vi "calibrate_tip.vi"() -> ()   [LabVIEW 2014]
uses:
  <vilib>/Analysis/Matrix/Datatypes/RealMatrix.ctl
  asap/labview/testing/calibration_task.ctl
  asap/labview/testing/cal_display_mode.ctl
  asap/labview/testing/probe_calibration.ctl
  <vilib>/Platform/TimedLoop/XDataNode/timing_clust.ctl
  <vilib>/Platform/TimedLoop/XDataNode/nitl_modes.ctl
  <vilib>/Platform/TimedLoop/XDataNode/wakeup.ctl
  testing/probe_point.ctl
  testing/pose_source.ctl
  <vilib>/gmath/NumericalOptimization/stopping criteria.ctl
  <vilib>/Analysis/baseanly.llb/A x Vector.vi
  initialization/micron_globals.vi
  <vilib>/gmath/NumericalOptimization/Downhill Simplex.vi
  <vilib>/Platform/TimedLoop/XDataNode/XDataNode.xnode
  <vilib>/Platform/TimedLoop/XDataNode/XDNodeRunTimeDep.lvlib
  <vilib>/Analysis/NI_AALBase.lvlib
  <vilib>/gmath/NI_Gmath.lvlib
  <vilib>/Analysis/Matrix/NI_Matrix.lvlib
panel:
  in  "Reference points 2":T1 format="%#.0f"
  in  "Valid override":bool
  out "status":bool
  out "Invalid data":bool
  out "Light triad error":dbl[](array[numeric]) format="%#.0f"
  out "Triad error":dbl
  in  "Save solution":bool
  in  "Clear all ref points":bool
  in  "Reference points":T1 format="%#.0f"
  in  "Calibration task":T2
  in  "Selector":bool[](array[boolean])
  out "Residuals":dbl[](array[numeric]) format="%#.0f"
  in  "Clear all":bool
  out "New point":dbl[](array[numeric]) format="%#.0f"
  in  "Save point":bool
  out "Number of poses":i32 format="%22.0f"
  out "Current point":dbl[](array[numeric]) format="%#.0f"
  out "RMS error":dbl format="%#22.0f"
  in  "Start calibration":bool
  out "Display mode":T3
  out "Light positions":sgl[][](array[numeric]) format="%#.2f"
  out "New light positions":sgl[][](array[numeric]) format="%#.2f"
  in  "Initialize light pos":bool
  in  "z offset":sgl=2262.0
  out "Calibration poses":dbl[][][](array[numeric])
  in  "stop":bool
  # "Point calibration (pivot)"
  # "(mm)"
  # "Position status"
  # "Three point calibrations"
  # "Handle"
  # "Tip"
  # "(mm)"
  # "(mm)"
  # "To calibrate the tip or RCM offset, position Micron in serveral different poses, keeping the desired calibration point (tip or RCM) fixed, but vary on all three of the rotational axes.  To record a pose, click \"Add pose\" or use the foot pedal to trigger a trace cycle.  The tool should be held still during the 0.2 sec data collection.  This can be done either fixtured or handheld, with or without cancellation. \n\nRecording least four poses is recommended.  RMS error should be <200 mm if fixtured, or ~ 1mm handheld.  You can use the \"Selector\" to remove poses with high residuals from the calibration.  Observe the sensitivity of  \"New point\" to adding and removing a pose from the estimate.  \"Save point\" stores this calibration into the running system.  To make it persistent, save it into the default configuration."
  # "Tip calibration requires a pivot calibration at each of three fiducial points on that part (either handle or tip.)  Fixture the probe, collect one pose, then press \"Initialize\".  Then do three pivot procedures (as for tip offset calibration.)  \"Save Point\" adds the measured location to the \"Reference Points\". Observe \"Triad error\" as a santity check. Finally, press \"Save solution.\"  Once tip lights have been calibrated and saved, the handle lights only need to be initialized (according to \"z offset\")."
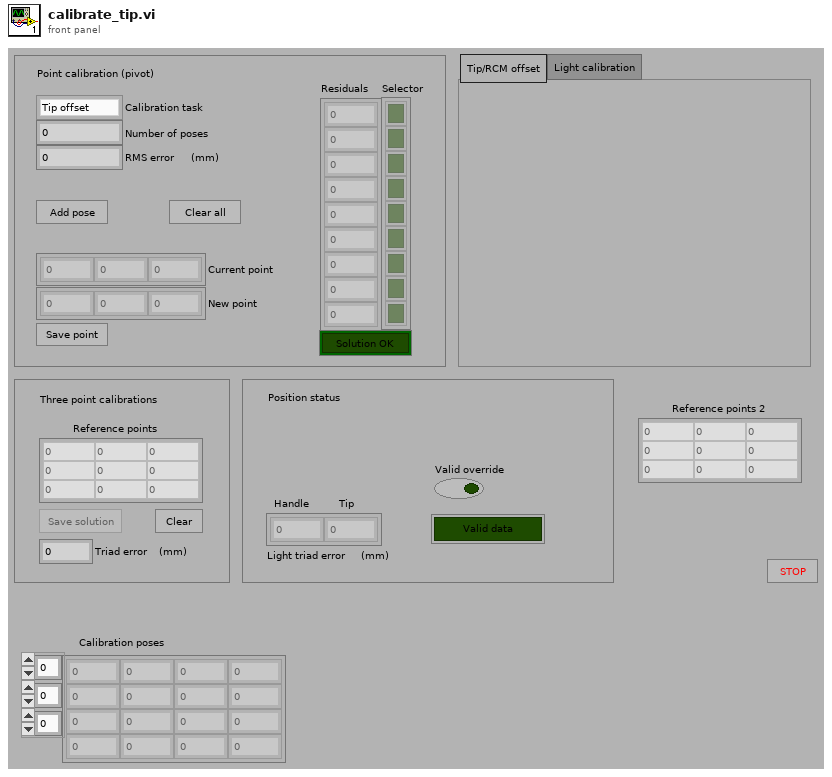
[diagram p1: front panel]
types:
  T1 = typedef "NI_Matrix.lvlib/RealMatrix.ctl" = dbl[][]
  T2 = typedef "calibration_task.ctl" = enum16{"Tip offset", "RCM offset", "Tip lights", "Handle lights"}
  T3 = typedef "cal_display_mode.ctl" = enum32{"Tip/RCM offset", "Light calibration"}
  T4 = enum16{"Off", "Step", "Sine", "Triangle", "Arbitrary"}
  T5 = typedef "probe_calibration.ctl" = sgl[][]
  T6 = typedef "NI_Gmath.lvlib/stopping criteria.ctl" = cluster{"function tolerance":dbl, "parameter tolerance":dbl, "max iterations":i32, "max function calls":i32, "gradient tolerance":dbl, "max time (sec)":dbl}
  T7 = typedef "pose_source.ctl" = enum16{"Output", "Handle", "Handle KF", "Goal", "Absolute"}
  T8 = typedef "probe_point.ctl" = enum16{"Position (tip)", "Position (RCM)", "Null pos (tip)", "Null pos (RCM)", "V limiter (tip)", "V Limiter (RCM)", "Goal filter (tip)", "Goal filter (RCM)", "Goal force (tip)", "Goal force (RCM)", "Goal (tip)", "Goal (RCM)", "Link pos 0", "Link pos 1", "KF link pos 0", "KF link pos 1", "Link rate 0", "Link rate 1", "Link residue 0", "Link residue 1", "Link goal 0", "Link goal 1", "Rate limit 0", "Rate limit 1", "Link error 0", "Link error 1", "Controller 0", "Controller 1", "Output 0", "Output 1", "Drive 0", "Drive 1", "Stimulus 0", "Stimulus 1", "Trace data 0", "Trace data 1", "Analog data 0", "Analog data 1", "Status flags", "Light 0", "Light 1", "Light 2", "Light 3", "Light 4", "Light 5", "Goal origin", "Goal rotation 0", "Goal rotation 1", "Goal rotation 2", "Output origin", "Output rotation 0", "Output rotation 1", "Output rotation 2", "Handle origin", "Handle rotation 0", "Handle rotation 1", "Handle rotation 2", "Handle position", "Handle velocity", "Handle acceleration", "Handle angles", "Handle angle rates", "Handle pos residue", "Handle angle residue", "Trace length"}
  T9 = typedef "XDNodeRunTimeDep.lvlib/timing_clust.ctl" = cluster{"Expected End [f-1]":u64, "Actual End [f-1]":u64, "Finished Late? [f-1]":bool, "Expected End [i-1]":u64, "Actual End [i-1]":u64, "Finished Late? [i-1]":bool, "Expected Start [i]":u64, "Actual Start [i]":u64, "Expected Start [f]":u64, "Actual Start [f]":u64, "Source Name":string, "Structure Name":string, "Period":i64, "Deadline":i64, "Offset":i64, "Start":i64, "Priority":i32, "Timeout":i32, "Mode":T10, "Wakeup Reason":T11, "Error":errorcluster, "Source Type":string, "Secondary Source Type":string, "Global End Time":u64, "Global Start Time":u64, "Frame Duration":u64, "Iteration Duration":u64, "Assigned CPU":i32, "I/O Scan Engine Mode":u32}
  T10 = typedef "XDNodeRunTimeDep.lvlib/nitl_modes.ctl" = enum32{"No Change", "Process missed periods, maintain original phase", "Discard missed periods, maintain original phase", "Process missed periods, ignore original phase", "Discard missed periods, ignore original phase"}
  T11 = typedef "XDNodeRunTimeDep.lvlib/wakeup.ctl" = enum32{"Normal", "Aborted", "Asynchronous wakeup", "Timing source error", "Timed loop error", "Timeout"}
  T12 = typedef "ui_override_opts.ctl" = cluster{"Triggering":bool, "Parameters":bool, "Stimulus":bool, "Calibration":bool, "Modes":bool}
  T13 = typedef "Micron params.ctl" = cluster{"Stimulus":T14, "Goal Filter A":T16, "Mode controls":T17, "Manipulator type":enum16{"Current piezo", "Voltage piezo"}, "Manipulator calibration":T18, "Network":T19, "Goal Filter B":T16, "Cancellation":T20, "Transition time":sgl, "Estimation":T22}
  T14 = typedef "stimulus.ctl" = cluster{"Type":enum16{"Off", "Step", "Sine", "Triangle", "Arbitrary"}, "Phase":dbl, "Amplitude":sgl[], "Injection point":T15, "Closed loop":bool, "Offset":sgl[], "Tip -> world":bool, "Frequency":dbl, "Length":dbl}
  T15 = typedef "injection_point.ctl" = enum16{"Total pose", "V limiter", "Goal ", "Link position", "KF link position", "Inverse kin", "Link goal", "Link error", "Controller", "Output", "Drive", "Light"}
  T16 = typedef "goal_loop_parms.ctl" = cluster{"Speedup max":sgl, "Speedup thresh":sgl, "Speedup nonlin":sgl, "Filters":cluster{"Lower Fc":sgl, "Lower Q":sgl, "Scale factor":sgl, "Upper Fc":sgl, "Upper Q":sgl, "V limit":sgl, "V limit range":sgl}[]}
  T17 = typedef "mode_conrols.ctl" = cluster{"Hold":bool, "Cancellation":bool, "Goal filter":bool, "Trigger":bool}
  T18 = typedef "manipulator_cal.ctl" = cluster{"Tool offsets":sgl[][], "Handle light calibration":T5, "Base pivots":sgl[][], "Output pivots":sgl[][], "Length center":sgl, "Workspace height":sgl[], "Workspace diameter":sgl[], "Stack travel":sgl, "Saturation pos":sgl, "Inverse filters":cluster{"filter structure":enum32{"IIR 2nd Order", "IIR 4th Order"}, "Reverse Coefficients":dbl[], "Forward Coefficients":dbl[]}[], "Strut length":sgl, "Tip light calibration":T5}
  T19 = typedef "network_params.ctl" = cluster{"Remote Host":string, "Send Status":bool, "Send Port":u16, "Recv Commands":bool, "Recv Port":u16}
  T20 = typedef "sq_control_params.ctl" = cluster{"KP":T21, "KI":sgl, "KD":T21, "Max vel":sgl, "Max acc":sgl, "Int error limit":sgl, "RCM gain":sgl, "Bypass":bool, "Degraded gain":sgl}
  T21 = typedef "decoupled_gain.ctl" = cluster{"XY":sgl, "Rxy":sgl, "Z":sgl, "Rz":sgl}
  T22 = typedef "estimation_controls.ctl" = cluster{"Link":cluster{"Measure noise":dbl[], "Process noise":dbl[], "Alt process noise":dbl[], "Alt turnoff cycles":i32, "Innovation limit":dbl[], "Residue threshold":dbl, "Enable":bool}, "Handle":cluster{"Measure noise":dbl[], "Process noise":dbl[], "State limits":dbl[], "Innovation limit":dbl[], "Prediction Lookahead":sgl, "Enable":bool}}
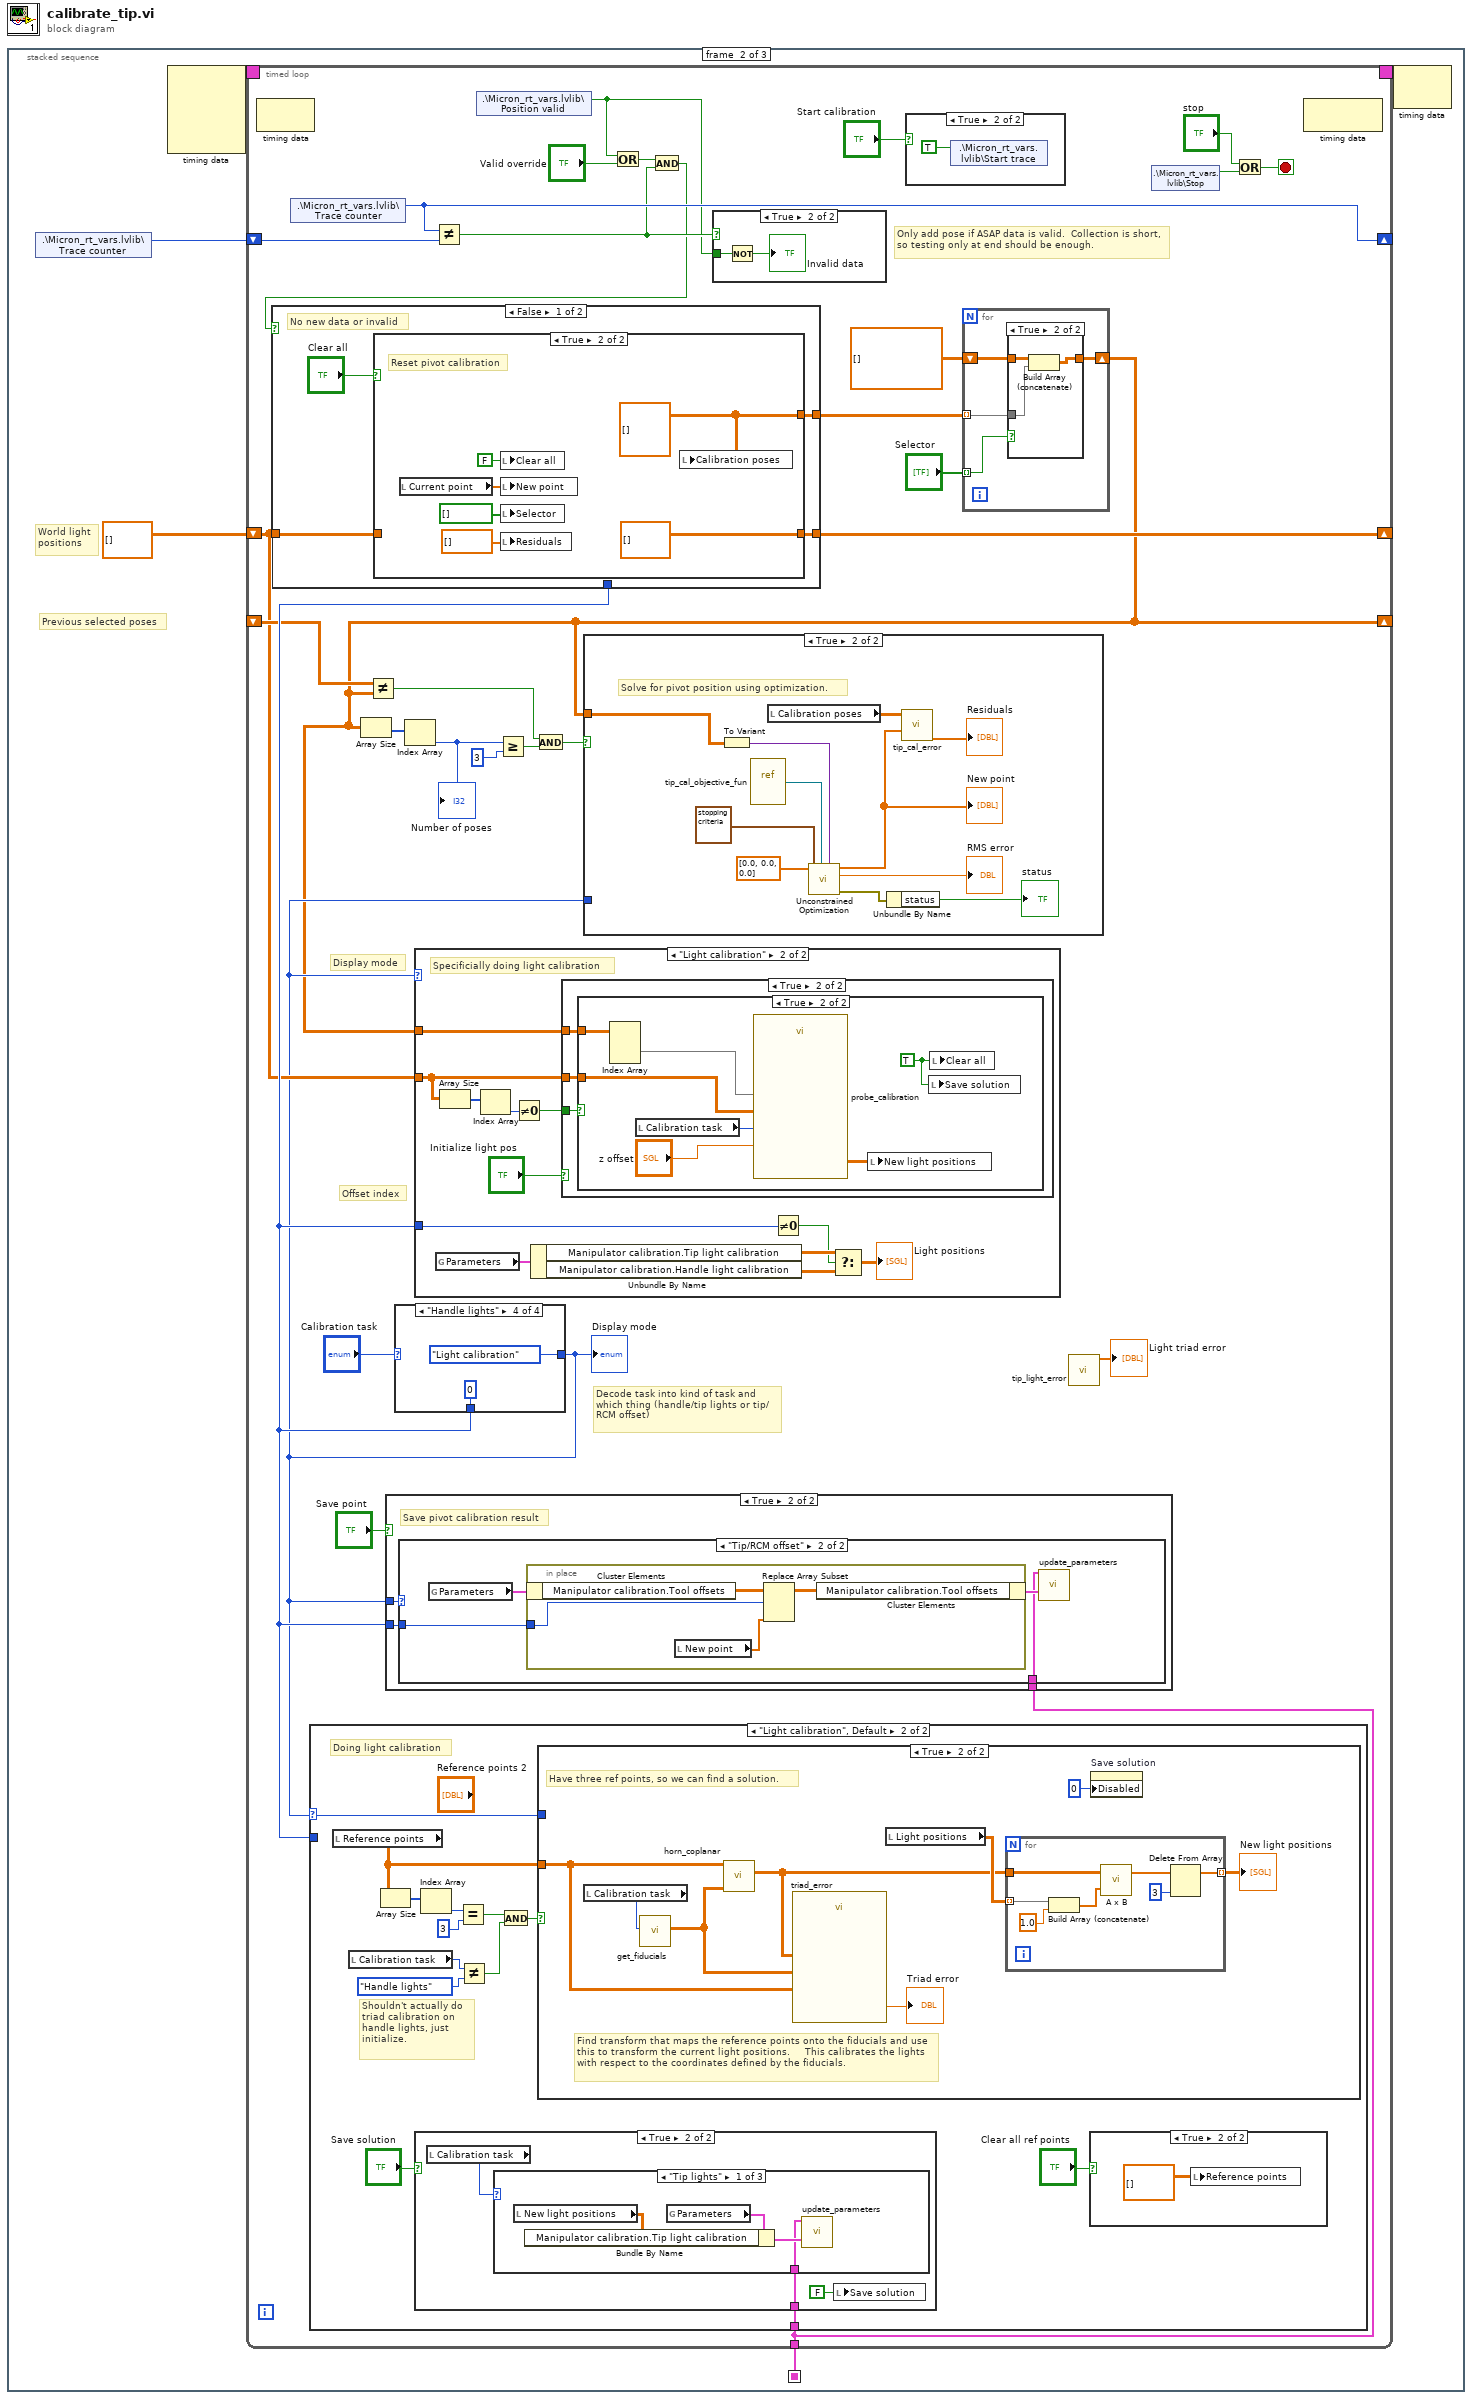
[diagram p0: block diagram]
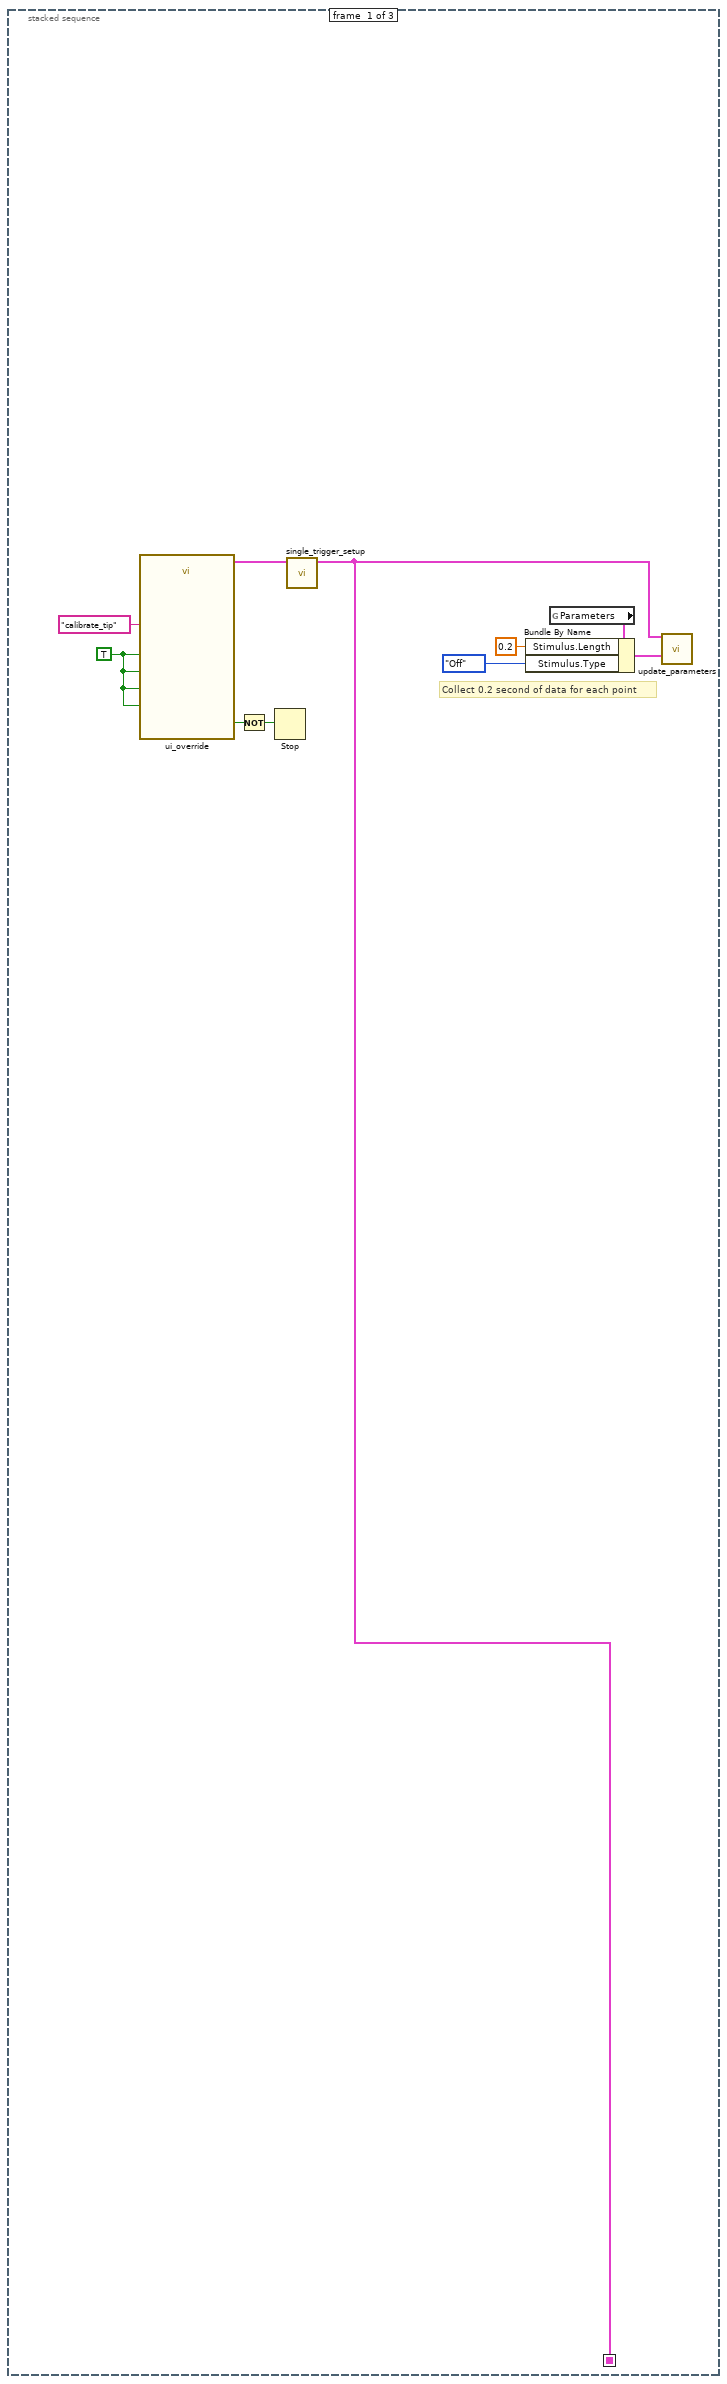
[diagram p2: hidden frame]
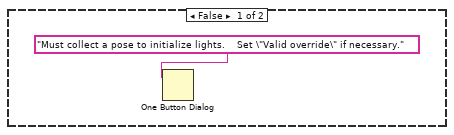
[diagram p6: hidden frame]
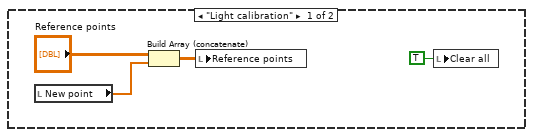
[diagram p8: hidden frame]
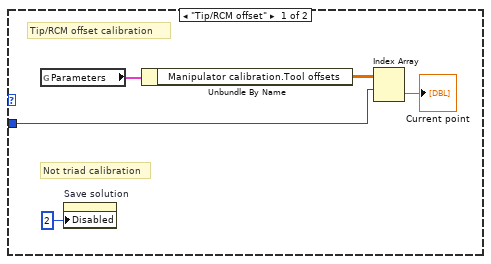
[diagram p9: hidden frame]
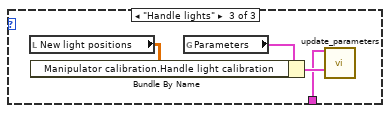
[diagram p12: hidden frame]
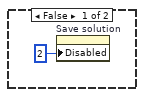
[diagram p14: hidden frame]
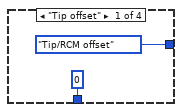
[diagram p15: hidden frame]
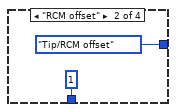
[diagram p16: hidden frame]
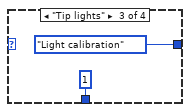
[diagram p17: hidden frame]
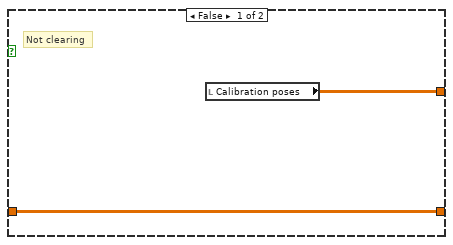
[diagram p20: hidden frame]
diagram:
  n1 = stacked-sequence {
    seq-local: [w4 _ _] -> [_ w11 _]
    frame #0 {
      w6 = TRUE ("All or nothing")
      # "Collect 0.2 second of data for each point"
      n2 = call "ui_override.vi"("Triggering"=w6, "VI name"="calibrate_tip", "Stimulus"=w6, "Calibration"=w6, "All or nothing"=w6) -> ("Override"=w5:T12, "Got all"=w2:bool)  [unwired: 8 in, 1 out]
      n3 = Not(x=w2) -> (.not. x?=w1:bool)
      n4 = Stop(stop? (T)=w1) -> ()
      n5 = call "single_trigger_setup.vi"("Override in"=w5) -> ("Override out"=w4:T12)  [unwired: 10 in]
      n6 = global read "micron_globals.vi" "Parameters"() -> (w9:T13)
      n7 = Bundle By Name(cluster=w9, "Stimulus.Length"=0.2, "Stimulus.Type"=T4."Off") -> (w10:T13)
      n8 = call "update_parameters.vi"("Modify"=w4, "Parameters"=w10) -> ()  [unwired: 12 in, 2 out]
    }
    frame #1 {
      # "World light\npositions"
      # "Previous selected poses"
      n9 = shared-variable ".\\Micron_rt_vars.lvlib\\Trace counter"() -> (w13:u32)  [unwired: 2 out]
      n10 = node-c288() -> (w15:T9)  [unwired: 4 out]
      n11 = timed-loop {
        timing: w15 -> [_]
        timing-out: [_] -> w14
        shift-right: [w42] -> _
        shift-left: w13 -> [w43]
        shift-right: [w23] -> _
        shift-left: _ -> [w30]
        shift-right: [w28] -> _
        shift-left: T5 [] ("Light positions") -> [w27]
        tunnel: w11 -> [w19]
        stop <- w22 stop-if-true
        # "Only add pose if ASAP data is valid.  Collection is short, so testing only at end should be enough."
        # "Decode task into kind of task and which thing (handle/tip lights or tip/RCM offset)"
        # "Offset index"
        # "Display mode"
        n12 = node-c288() -> ()  [unwired: 2 out]
        n13 = shared-variable ".\\Micron_rt_vars.lvlib\\Trace counter"() -> (w42:u32)  [unwired: 2 out]
        n14 = case shown="\"Handle lights\"" "Calibration task" {
          tunnel: [cal_display_mode."Tip/RCM offset" ("Display mode") cal_display_mode."Tip/RCM offset" ("Display mode") cal_display_mode."Light calibration" ("Display mode") cal_display_mode."Light calibration" ("Display mode")] -> w24
          tunnel: [0 ("disabled index (col)") 1 ("disabled index (col)") 1 ("disabled index (col)") 0 ("disabled index (col)")] -> w45
          frame "Tip offset" {
          }
          frame "RCM offset" {
          }
          frame "Tip lights" {
          }
          frame "Handle lights" {
          }
        }
        "Display mode" <- w24
        n15 = case shown="\"Light calibration\", Default" w24 {
          selector: w24 -> [_ w97]
          tunnel: w45 -> [w87 _]
          tunnel: w19 -> [_ w91]
          frame "Tip/RCM offset" {
            # "Tip/RCM offset calibration"
            # "Not triad calibration"
            n16 = global read "micron_globals.vi" "Parameters"() -> (w89:T13)
            n17 = property on="Save solution" class="Bool (strict)"("Disabled"=u8 2) -> ()  [unwired: 2 in, 2 out]
            n18 = Unbundle By Name(w89) -> ("Manipulator calibration.Tool offsets"=w88:sgl[][])
            n19 = Index Array(array=w88, index (row)=w87) -> (element=→"Current point":sgl[])  [unwired: 1 in]
          }
          frame "Light calibration", Default {
            # "Shouldn't actually do\ntriad calibration on\nhandle lights, just \ninitialize."
            # "Doing light calibration"
            n20 = local read "Reference points"() -> (w100:T1)
            n21 = local read "Calibration task"() -> (w94:T2)
            n22 = Array Size(array=w100) -> (size(s)=w103:i32[])
            n23 = case shown="True" "Save solution" {
              tunnel: w91 -> [_ w104]
              frame False {
              }
              frame True {
                n24 = local read "Calibration task"() -> (w106:T2)
                n25 = case shown="\"Tip lights\"" w106 {
                  tunnel: w104 -> [w107 _ w111]
                  frame "Tip lights" {
                    n26 = local read "New light positions"() -> (w108:sgl[][])
                    n27 = global read "micron_globals.vi" "Parameters"() -> (w109:T13)
                    n28 = Bundle By Name(cluster=w109, "Manipulator calibration.Tip light calibration"=w108) -> (w110:T13)
                    n29 = call "update_parameters.vi"("Modify"=w107, "Parameters"=w110) -> ()  [unwired: 12 in, 2 out]
                  }
                  frame "RCM offset", Default {
                    # "This is handled by \"Save point\""
                  }
                  frame "Handle lights" {
                    n30 = local read "New light positions"() -> (w112:sgl[][])
                    n31 = global read "micron_globals.vi" "Parameters"() -> (w113:T13)
                    n32 = Bundle By Name(cluster=w113, "Manipulator calibration.Handle light calibration"=w112) -> (w114:T13)
                    n33 = call "update_parameters.vi"("Modify"=w111, "Parameters"=w114) -> ()  [unwired: 12 in, 2 out]
                  }
                }
                n34 = local write "Save solution"(FALSE ("Save solution")) -> ()
              }
            }
            n35 = Index Array(array=w103) -> (element=w102:i32)  [unwired: 1 in]
            n36 = Equal?(x=w102, y=3) -> (x = y?=w96:bool)
            n37 = Not Equal?(x=w94, y=calibration_task."Handle lights" ("Calibration task")) -> (x != y?=w92:bool)
            n38 = And(x=w96, y=w92) -> (x .and. y?=w95:bool)
            n39 = case shown="True" w95 {
              tunnel: w100 -> [_ w124]
              tunnel: w97 -> [_ _]
              frame False {
                n40 = property on="Save solution" class="Bool (strict)"("Disabled"=u8 2) -> ()  [unwired: 2 in, 2 out]
              }
              frame True {
                # "Find transform that maps the reference points onto the fiducials and use this to transform the current light positions.     This calibrates the lights with respect to the coordinates defined by the fiducials."
                # "Have three ref points, so we can find a solution."
                n41 = local read "Calibration task"() -> (w117:T2)
                n42 = call "get_fiducials.vi"("Calibration task"=w117) -> ("Fiducial points"=w119:T1)  [unwired: 10 in]
                n43 = call "horn_coplanar.vi"("Right points"=w119, "Left points"=w124) -> ("LR transform"=w120:T1)  [unwired: 9 out]
                n44 = call "triad_error.vi"("Measured positions"=w124, "Measure transform"=w120, "Calibrated positions"=w119) -> ("RMS error"=→"Triad error":dbl)  [unwired: 7 in, 1 out]
                n45 = local read "Light positions"() -> (w122:sgl[][])
                n46 = for {
                  tunnel: w120 -> [w131]
                  tunnel: w122 -> [w128] mode=indexing
                  tunnel: [w125] -> w121 mode=indexing
                  n47 = Build Array (concatenate)(w128, 1.0 ("disabled index (col)")) -> (w129:dbl[])
                  n48 = call-poly <vilib>:"A x B.vi"("Vector"=w129, "A"=w131) -> ("A x Vector"=w127:dbl[])  [unwired: 1 out]
                  n49 = Delete From Array(array=w127, index=3) -> (array with subset deleted=w125:dbl[])  [unwired: 1 in, 1 out]
                }
                "New light positions" <- w121
                n50 = property on="Save solution" class="Bool (strict)"("Disabled"=u8 0) -> ()  [unwired: 2 in, 2 out]
              }
            }
            n51 = case shown="True" "Clear all ref points" {
              frame False {
              }
              frame True {
                n52 = local write "Reference points"(T1 [] ("Marked points")) -> ()
              }
            }
          }
        }
        n53 = case shown="True" "Save point" {
          tunnel: w24 -> [_ w73]
          tunnel: w45 -> [_ w72]
          tunnel: w19 -> [_ w71]
          frame False {
          }
          frame True {
            # "Save pivot calibration result"
            n54 = case shown="\"Tip/RCM offset\"" w73 {
              tunnel: w72 -> [_ w80]
              tunnel: w71 -> [_ w78]
              frame "Light calibration" {
                n55 = local read "New point"() -> (w76:dbl[])
                n56 = Build Array (concatenate)("Reference points", w76) -> (w77:T1)
                n57 = local write "Reference points"(w77) -> ()
                n58 = local write "Clear all"(TRUE ("Clear all")) -> ()
              }
              frame "Tip/RCM offset" {
                n59 = global read "micron_globals.vi" "Parameters"() -> (w81:T13)
                n60 = in-place {
                  in-place-border: w80 -> [w83]
                  n61 = in-place-cluster #1(w81) -> ("Manipulator calibration.Tool offsets"=w85:sgl[][])
                  n62 = local read "New point"() -> (w82:dbl[])
                  n63 = Replace Array Subset(array=w85, new element=w82, index (row)=w83) -> (w84:sgl[][])  [unwired: 1 in]
                  n64 = in-place-cluster #1("Manipulator calibration.Tool offsets"=w84) -> (w79:T13)
                }
                n65 = call "update_parameters.vi"("Modify"=w78, "Parameters"=w79) -> ()  [unwired: 12 in, 2 out]
              }
            }
          }
        }
        n66 = Not Equal?(x=w42, y=w43) -> (x != y?=w26:bool)
        n67 = shared-variable ".\\Micron_rt_vars.lvlib\\Position valid"() -> (w17:bool)  [unwired: 2 out]
        n68 = Or(x=w17, y="Valid override") -> (x .or. y?=w16:bool)
        n69 = And(x=w16, y=w26) -> (x .and. y?=w25:bool)
        n70 = case shown="False" w25 {
          tunnel: [w162 w174] -> w34
          tunnel: w45 -> [_ w176]
          tunnel: [w161 w175] -> w28
          tunnel: w27 -> [w160 _]
          frame False {
            # "No new data or invalid"
            n71 = case shown="True" "Clear all" {
              tunnel: [w163 w165] -> w162
              tunnel: [w164 T5 [] ("Light positions")] -> w161
              tunnel: w160 -> [w164 _]
              frame False {
                # "Not clearing"
                n72 = local read "Calibration poses"() -> (w163:dbl[][][])
              }
              frame True {
                w165 = dbl[][][] [] ("Decimated pose (manipulator)")
                # "Reset pivot calibration"
                n73 = local read "Current point"() -> (w168:dbl[])
                n74 = local write "Clear all"(FALSE ("Clear all")) -> ()
                n75 = local write "New point"(w168) -> ()
                n76 = local write "Selector"(bool[] [] ("Selector")) -> ()
                n77 = local write "Residuals"(dbl[] [] ("Residuals")) -> ()
                n78 = local write "Calibration poses"(w165) -> ()
              }
            }
          }
          frame True {
            # "Always get output pose, even for\nhandle light initialization."
            # "Decimate to single record"
            # "New valid data"
            n79 = call "trace_data.vi"("Decimate"=-1) -> ("Decimated trace"=w182:sgl[][][])  [unwired: 8 in, 2 out]
            n80 = Index Array(array=w182) -> (element=w180:sgl[][])  [unwired: 3 in]
            n81 = Array Subset(array=w180, index (row)=probe_point."Light 0" ("Origin index"), length (row)=6 ("length")) -> (w177:sgl[][])  [unwired: 2 in]
            n82 = local read "Calibration poses"() -> (w173:dbl[][][])
            n83 = local read "Selector"() -> (w185:bool[])
            n84 = call "get_pose.vi"("Selector"=pose_source."Output", "Input Trace"=w180) -> ("Pose"=w181:T1)  [unwired: 9 in]
            n85 = call "get_lights.vi"("Selector"=w176, "ASAP data"=w177) -> ("Light positions"=w175:T5)  [unwired: 9 in]
            n86 = Build Array (concatenate)(w185, TRUE ("Reoptimize")) -> (w184:bool[])
            n87 = Build Array (concatenate)(w173, w181) -> (w174:dbl[][][])
            "Calibration poses" <- w174
            n88 = local write "Selector"(w184) -> ()
          }
        }
        n89 = case shown="True" w26 {
          tunnel: w17 -> [_ w47]
          frame False {
          }
          frame True {
            n90 = Not(x=w47) -> (.not. x?=→"Invalid data":bool)
          }
        }
        n91 = case shown="True" "Start calibration" {
          frame False {
          }
          frame True {
            n92 = shared-variable ".\\Micron_rt_vars.lvlib\\Start trace"(TRUE ("Start trace")) -> ()  [unwired: 2 out]
          }
        }
        n93 = for {
          tunnel: w34 -> [w142] mode=indexing
          tunnel: "Selector" -> [w143] mode=indexing
          shift-right: [w140] -> w23
          shift-left: dbl[][][] [] ("Calibration point pose") -> [w141]
          n94 = case shown="True" w143 {
            tunnel: w142 -> [_ w147]
            tunnel: w141 -> [w144 w146]
            tunnel: [w144 w145] -> w140
            frame False {
            }
            frame True {
              n95 = Build Array (concatenate)(w146, w147) -> (w145:dbl[][][])
            }
          }
        }
        n96 = Array Size(array=w23) -> (size(s)=w40:i32[])
        n97 = Not Equal?(x=w30, y=w23) -> (x != y?=w32:bool)
        n98 = Index Array(array=w40) -> (element=w39:i32)  [unwired: 1 in]
        "Number of poses" <- w39
        n99 = case shown="\"Light calibration\"" w24 {
          tunnel: w27 -> [_ w54]
          tunnel: w45 -> [_ w52]
          tunnel: w23 -> [_ w50]
          frame "Tip/RCM offset" {
          }
          frame "Light calibration" {
            # "Specificially doing light calibration"
            n100 = global read "micron_globals.vi" "Parameters"() -> (w59:T13)
            n101 = Array Size(array=w54) -> (size(s)=w56:i32[])
            n102 = Index Array(array=w56) -> (element=w55:i32)  [unwired: 1 in]
            n103 = Not Equal To 0?(x=w55) -> (x != 0?=w48:bool)
            n104 = Unbundle By Name(w59) -> ("Manipulator calibration.Tip light calibration"=w58:T5, "Manipulator calibration.Handle light calibration"=w57:T5)
            n105 = case shown="True" "Initialize light pos" {
              tunnel: w54 -> [_ w62]
              tunnel: w50 -> [_ w61]
              tunnel: w48 -> [_ w60]
              frame False {
              }
              frame True {
                n106 = case shown="True" w60 {
                  tunnel: w62 -> [_ w70]
                  tunnel: w61 -> [_ w65]
                  frame False {
                    n107 = One Button Dialog(message="Must collect a pose to initialize lights.    Set \"Valid override\" if necessary.") -> ()  [unwired: 1 in, 1 out]
                  }
                  frame True {
                    w68 = TRUE ("Clear all")
                    n108 = Index Array(array=w65) -> (element=w64:dbl[][])  [unwired: 3 in]
                    n109 = local read "Calibration task"() -> (w67:T2)
                    n110 = call "probe_calibration.vi"("z offset"="z offset", "Calibration task"=w67, "World light positions"=w70, "Output pose"=w64) -> ("Probe calibration"=w69:T5)  [unwired: 7 out]
                    n111 = local write "New light positions"(w69) -> ()
                    n112 = local write "Save solution"(w68) -> ()
                    n113 = local write "Clear all"(w68) -> ()
                  }
                }
              }
            }
            n114 = Not Equal To 0?(x=w52) -> (x != 0?=w53:bool)
            n115 = Select(t=w58, s=w53, f=w57) -> (s? t:f=→"Light positions":T5)
          }
        }
        n116 = Greater Or Equal?(x=w39, y=3) -> (x >= y?=w37:bool)
        n117 = And(x=w32, y=w37) -> (x .and. y?=w41:bool)
        n118 = case shown="True" w41 {
          tunnel: w23 -> [_ w158]
          tunnel: w24 -> [_ _]
          frame False {
          }
          frame True {
            # "Solve for pivot position using optimization."
            n119 = To Variant(anything=w158) -> (Variant=w155:variant)
            n120 = vi-ref "tip_cal_objective_fun.vi"() -> (w156:refnum<vi>)
            n121 = local read "Calibration poses"() -> (w148:dbl[][][])
            n122 = call-poly <vilib>:"Unconstrained Optimization.vi"("function data"=w155, "objective function"=w156, "stopping criteria"=T6 {"function tolerance"=1e-06, "parameter tolerance"=1e-06, "max iterations"=1000, "max function calls"=2000, "gradient tolerance"=1e-06, "max time (sec)"=-1.0} ("Stopping criteria"), "start"=dbl[] [0.0, 0.0, 0.0]) -> ("error out"=w150:errorcluster, "f(minimum)"=→"RMS error":dbl, "minimum"=w152:dbl[])  [unwired: 1 in, 4 out]
            "New point" <- w152
            n123 = Unbundle By Name(w150) -> ("status"=→"status":bool)
            n124 = call "tip_cal_error.vi"("X"=w152, "Calibration point pose"=w148) -> ("Residuals"=→"Residuals":dbl[])  [unwired: 1 in, 8 out]
          }
        }
        n125 = call "tip_light_error.vi"() -> ("RMS error"=→"Light triad error":dbl[])  [unwired: 11 out]
        n126 = shared-variable ".\\Micron_rt_vars.lvlib\\Stop"() -> (w21:bool)  [unwired: 1 in, 1 out]
        n127 = Or(x="stop", y=w21) -> (x .or. y?=w22:bool)
        n128 = node-c288() -> ()  [unwired: 2 out]
      }
      n129 = node-c288(w14) -> ()  [unwired: 1 out]
    }
    frame #2 {
      n130 = call "ui_override.vi"("VI name"="calibrate_tip") -> ()  [unwired: 12 in, 3 out]
    }
  }
